vi "startThread.vi"(0 "HGF_ThreadPool_Reference":refnum<class "HGF_Reference.lvclass">, 3 "timeout in ms (-1)":i32=-1, 5 "error in (no error)":errorcluster) -> (14 "HGF_ThreadPool_Reference":refnum<class "HGF_Reference.lvclass">, 17 "got object?":bool, 19 "error out":errorcluster)   [LabVIEW 2014, in "HGF_BaseClasses.lvlib" / "HGF_ThreadWorker.lvclass"]
doc: "Start a new thread.\n\n<b>Attention:</b> This VI should be call from HGF_ThreadPool.startThread.vi only!"
uses:
  HGF_ThreadWorker.lvclass
  HGF_ThreadPool/HGF_ThreadPool.lvclass
  HGF_Reference/HGF_Reference.lvclass
  HGF_Auxiliary/HGF_Auxiliary.lvlib
  callThread.vi
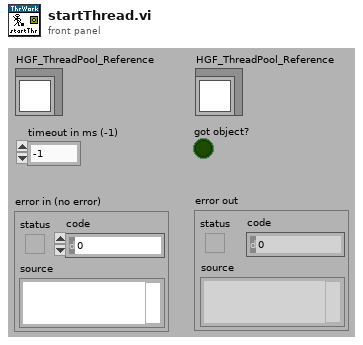
[diagram p1: front panel]
types:
  T1 = enum32{"invalid app kind", "Development System", "Run Time System", "Student Edition", "Embedded LabVIEW", "Evaluation", "Custom"}
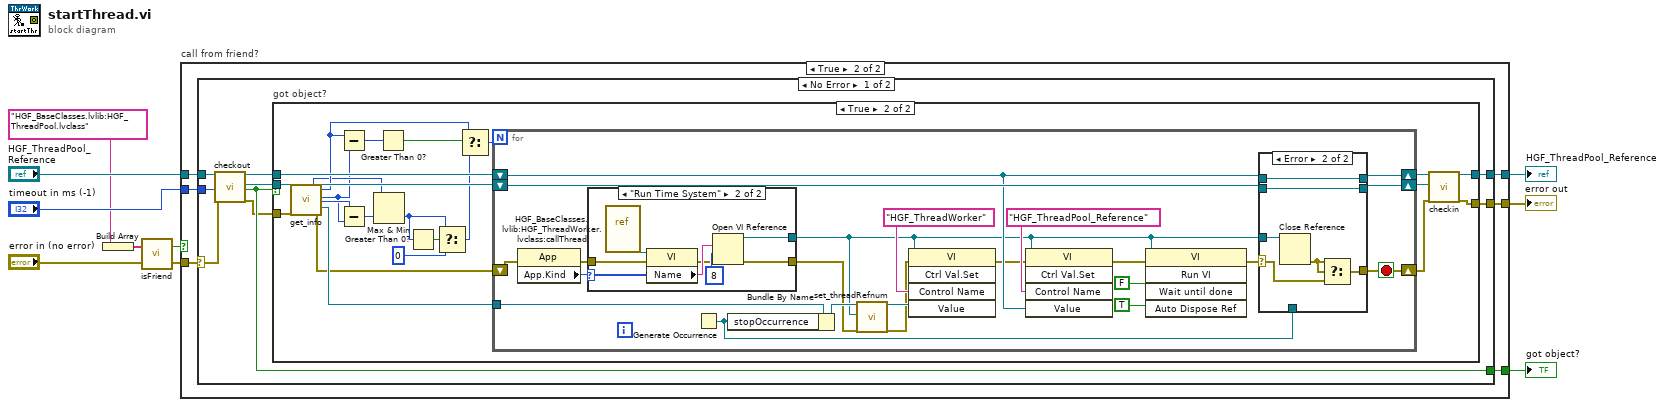
[diagram p0: block diagram]
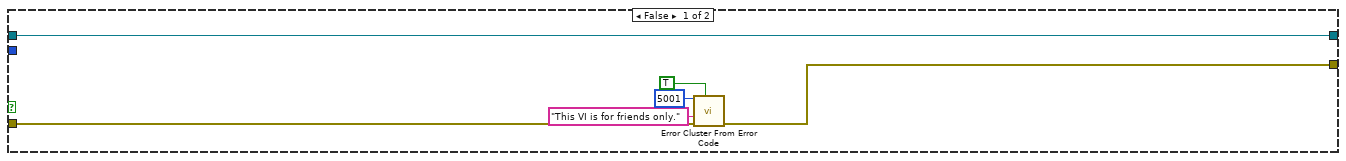
[diagram p2: hidden frame]
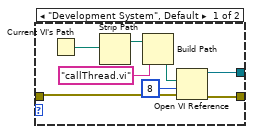
[diagram p4: hidden frame]
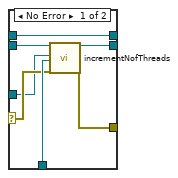
[diagram p5: hidden frame]
diagram:
  n1 = Build Array("HGF_BaseClasses.lvlib:HGF_ThreadPool.lvclass" ("y")) -> (w1:string[])
  n2 = call "isFriend.vi"("error in (no error)"="error in (no error)", "Friends"=w1) -> ("error out"=w4:errorcluster, "isFriend?"=w3:bool)
  n3 = case "call from friend?" shown="True" w3 {
    tunnel: [w12 w22] -> w10
    tunnel: w4 -> [w13 w21]
    tunnel: "HGF_ThreadPool_Reference" -> [w16 w20]
    tunnel: [w16 w19] -> w8
    tunnel: "timeout in ms (-1)" -> [_ w18]
    tunnel: [_ w17] -> w6
    frame False {
      n4 = call <vilib>:"Error Cluster From Error Code.vi"("show call chain? (False)"=TRUE, "error in (no error)"=w13, "error message (\"\")"="This VI is for friends only." ("error message (\"\")"), "error code (0)"=5001) -> ("error out"=w12:errorcluster)  [unwired: 5 out]
    }
    frame True {
      n5 = case shown="No Error" w21 {
        selector: w21 -> [w24 w108]
        tunnel: [w31 w108] -> w22
        tunnel: w20 -> [w30 w107]
        tunnel: [w27 w107] -> w19
        tunnel: w18 -> [w28 _]
        tunnel: [w25 _] -> w17
        frame No Error {
          n6 = call "checkout.vi"("HGF_ThreadPool_Reference"=w30, "timeout in ms (-1)"=w28, "error in (no error)"=w24) -> ("dup HGF_ThreadPool_Reference"=w29:refnum<class "HGF_Reference.lvclass">, "HGF_ThreadPool"=w26:refnum<class "HGF_ThreadPool.lvclass">, "got object?"=w25:bool, "error out"=w23:errorcluster)  [unwired: 13 out]
          n7 = case "got object?" shown="True" w25 {
            tunnel: [w33 w34] -> w31
            tunnel: w29 -> [w32 w49]
            tunnel: [w32 w56] -> w27
            tunnel: w23 -> [w33 w54]
            tunnel: w26 -> [_ w55]
            frame False {
            }
            frame True {
              n8 = call "get_info.vi"("HGF_ThreadPool"=w55, "error in (no error)"=w54) -> ("incThreads"=w42:i32, "dup HGF_ThreadPool"=w52:refnum<class "HGF_ThreadPool.lvclass">, "initialNofThreads"=w46:i32, "nofThreads"=w37:i32, "maxNofThreads"=w38:i32, "HGF_ThreadWorker"=w53:refnum<class "HGF_ThreadWorker.lvclass">, "error out"=w36:errorcluster)  [unwired: 11 out]
              n9 = Subtract(x=w46, y=w37) -> (x-y=w51:i32)
              n10 = Subtract(x=w38, y=w37) -> (x-y=w41:i32)
              n11 = Max & Min(x=w42, y=w41) -> (min(x,y)=w40:i32)  [unwired: 1 out]
              n12 = Greater Than 0?(x=w51) -> (x > 0?=w47:bool)
              n13 = Greater Than 0?(x=w40) -> (x > 0?=w39:bool)
              n14 = Select(t=w40, s=w39, f=0) -> (s? t:f=w44:i32)
              n15 = Select(t=w46, s=w47, f=w44) -> (s? t:f=w45:i32)
              n16 = for {
                N: w45 -> [_]
                tunnel: w53 -> [w68]
                shift-right: [w72] -> w50
                shift-left: w49 -> [w71]
                shift-right: [w70] -> w48
                shift-left: w52 -> [w73]
                shift-right: [w69] -> w35
                shift-left: w36 -> [w58]
                stop <- w69 stop-if-true
                n17 = property class="App"(error in=w58) -> (error out=w57:errorcluster, "App.Kind"=w59:T1)  [unwired: 1 in, 1 out]
                n18 = case shown="\"Run Time System\"" w59 {
                  tunnel: w57 -> [w81 w90]
                  tunnel: [w80 w88] -> w65
                  tunnel: [w79 w87] -> w60
                  frame "Development System", Default {
                    n19 = Current VI's Path() -> (path=w84:path)
                    n20 = Strip Path(path=w84) -> (stripped path=w83:path)  [unwired: 1 out]
                    n21 = Build Path(base path=w83, name or relative path="callThread.vi") -> (appended path=w82:path)
                    n22 = Open VI Reference(vi path=w82, options=8, error in (no error)=w81) -> (vi reference=w79:refnum<vi>, error out=w80:errorcluster)  [unwired: 1 in, 2 out]
                  }
                  frame "Run Time System" {
                    n23 = vi-ref "HGF_BaseClasses.lvlib:HGF_ThreadWorker.lvclass:callThread.vi"() -> (w92:refnum<vi>)
                    n24 = property class="VI"(reference=w92, error in=w90) -> (error out=w89:errorcluster, "Name"=w91:string)  [unwired: 1 out]
                    n25 = Open VI Reference(vi path=w91, options=8, error in (no error)=w89) -> (vi reference=w87:refnum<vi>, error out=w88:errorcluster)  [unwired: 1 in, 2 out]
                  }
                }
                n26 = Generate Occurrence() -> (w66:refnum<k4>)
                n27 = Bundle By Name(cluster=w68, "stopOccurrence"=w66) -> (w67:refnum<class "HGF_ThreadWorker.lvclass">)
                n28 = call "set_threadRefnum.vi"("HGF_ThreadWorker"=w67, "threadRefnum"=w60, "error in (no error)"=w65) -> ("dup HGF_ThreadWorker"=w74:refnum<class "HGF_ThreadWorker.lvclass">, "error out"=w62:errorcluster)  [unwired: 15 out]
                n29 = invoke class="VI" method="Ctrl Val.Set"(reference=w60, error in=w62, "Control Name"="HGF_ThreadWorker", "Value"=w74) -> (error out=w61:errorcluster)  [unwired: 1 in, 4 out]
                n30 = invoke class="VI" method="Ctrl Val.Set"(reference=w60, error in=w61, "Control Name"="HGF_ThreadPool_Reference", "Value"=w71) -> (error out=w63:errorcluster)  [unwired: 1 in, 4 out]
                n31 = invoke class="VI" method="Run VI"(reference=w60, error in=w63, "Wait until done"=FALSE ("Wait Until Done"), "Auto Dispose Ref"=TRUE ("Auto Dispose Reference")) -> (error out=w64:errorcluster)  [unwired: 1 in, 4 out]
                n32 = case shown="Error" w64 {
                  selector: w64 -> [w95 w103]
                  tunnel: w60 -> [w94 w106]
                  tunnel: [w99 w104] -> w69
                  tunnel: w73 -> [w100 w101]
                  tunnel: [w98 w102] -> w72
                  tunnel: w71 -> [w98 w102]
                  tunnel: [w97 w101] -> w70
                  tunnel: w66 -> [w96 _]
                  frame No Error {
                    n33 = call "incrementNofThreads.vi"("HGF_ThreadPool"=w100, "threadRef"=w94, "stopOccurrence"=w96, "error in (no error)"=w95) -> ("dup HGF_ThreadPool"=w97:refnum<class "HGF_ThreadPool.lvclass">, "error out"=w99:errorcluster)  [unwired: 14 out]
                  }
                  frame Error {
                    n34 = Close Reference(reference=w106) -> (error out=w105:errorcluster)  [unwired: 1 in]
                    n35 = Select(t=w105, s=w105, f=w103) -> (s? t:f=w104:errorcluster)
                  }
                }
              }
              n36 = call "checkin.vi"("HGF_Reference"=w50, "Object"=w48, "error in (no error)"=w35) -> ("dup HGF_Reference"=w56:refnum<class "HGF_Reference.lvclass">, "error out"=w34:errorcluster)  [unwired: 1 in, 14 out]
            }
          }
        }
        frame Error {
        }
      }
    }
  }
  "error out" <- w10
  "HGF_ThreadPool_Reference" <- w8
  "got object?" <- w6
